vi "emi_Get Status Loop.vi"(5 "Loop ID in":u16, 9 "error in (no error)":errorcluster) -> (6 "Loop ID out":u16, 8 "Loop Running Out":bool, 10 "error out":errorcluster)   [LabVIEW 2010]
doc: "Retreive the execution state of the loop designated by Index. Used to syncronice different loops in teh same master loop"
uses:
  Private/_emi_Loop control int action.ctl
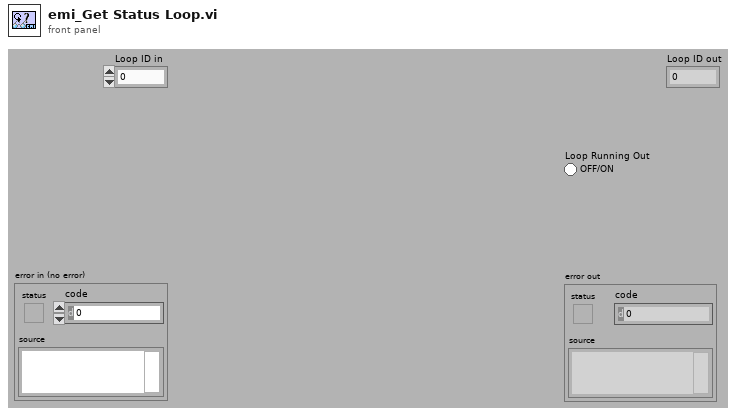
[diagram p1: front panel]
types:
  T1 = typedef "_emi_Loop control int action.ctl" = enum16{"Init index", "Get index", "Set index", "Get Size"}
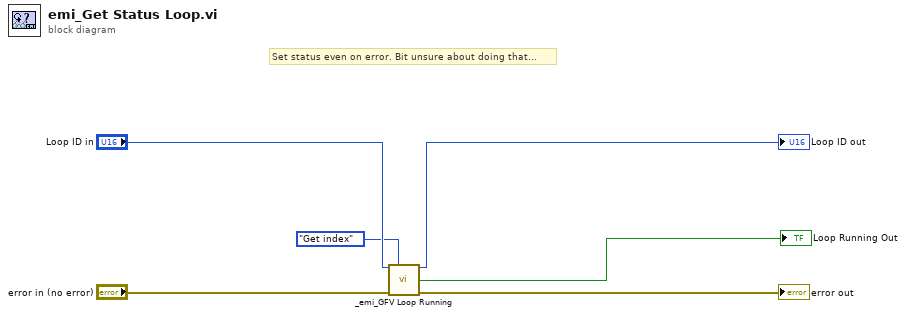
[diagram p0: block diagram]
diagram:
  # "Set status even on error. Bit unsure about doing that..."
  n1 = call "_emi_GFV Loop Running.vi"("Loop Index/Numb"="Loop ID in", "Action(Get Index)"=_emi_Loop_control_int_action."Get index", "error in (no error)"="error in (no error)") -> ("Index out"=→"Loop ID out":u16, "Loop Running Out"=→"Loop Running Out":bool, "error out"=→"error out":errorcluster)  [unwired: 9 in, 1 out]
